vi "Horizontal Bar Get Picure by Enum.vi"(11 "Type":T1) -> (3 "value":picture)   [LabVIEW 2020, in "BetterDragAndDrop.lvlib" / "BetterHorizontalBar.lvclass"]
uses:
  BetterHorizontalBar.lvclass
  Horizontal Bar Enumeration.ctl
  Horizontal Bar Map.ctl
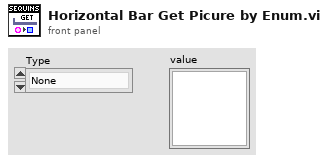
[diagram p1: front panel]
types:
  T1 = typedef "BetterDragAndDrop.lvlib/BetterHorizontalBar.lvclass/Horizontal Bar Enumeration.ctl" = enum16{"None", "only bar", "tilda up"}
  T2 = typedef "BetterDragAndDrop.lvlib/BetterHorizontalBar.lvclass/Horizontal Bar Map.ctl" = map{T1, picture}
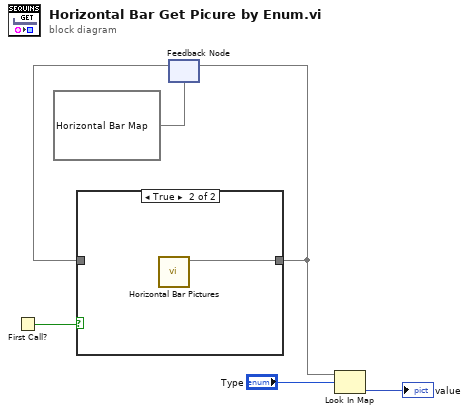
[diagram p0: block diagram]
diagram:
  n1 = First Call?() -> (First Call?: T/F=w6:bool)
  n2 = feedback #1(T2 {} ("Horizontal bar map")) -> (w5:T2)
  n3 = case shown="True" w6 {
    tunnel: [w7 w8] -> w3
    tunnel: w5 -> [w7 _]
    frame False {
    }
    frame True {
      n4 = call "Horizontal Bar Pictures.vi"() -> ("Horizontal bar map"=w8:T2)  [unwired: 11 in]
    }
  }
  n5 = feedback-in #1(w3) -> ()
  n6 = Look In Map(map=w3, key="Type") -> (value=→"value":picture)  [unwired: 1 in, 1 out]
